vi "New JSON Numeric.vi"(8 "error in (no error)":errorcluster, 10 "value":dbl) -> (0 "error out":errorcluster, 3 "JSON Value out":refnum<class "JSON Value.lvclass">)   [LabVIEW 2016, in "JSON Value.lvclass"]
doc: "Create a new JSON Numeric with the given value."
uses:
  JSON Value.lvclass
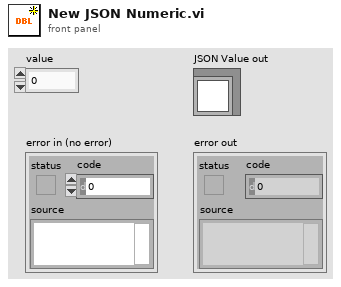
[diagram p1: front panel]
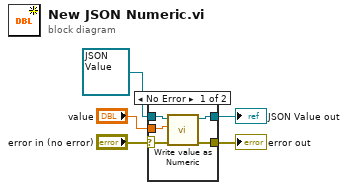
[diagram p0: block diagram]
diagram:
  n1 = case shown="No Error" "error in (no error)" {
    selector: "error in (no error)" -> [w8 w12]
    tunnel: [w10 w12] -> w4
    tunnel: [w6 w11] -> w3
    tunnel: refnum<class "JSON Value.lvclass"> refnum ("JSON out") -> [w9 w11]
    tunnel: "value" -> [w7 _]
    frame No Error {
      n2 = call "Write value as Numeric.vi"("error in (no error)"=w8, "value"=w7, "JSON Value in"=w9) -> ("error out"=w10:errorcluster, "JSON Value out"=w6:refnum<class "JSON Value.lvclass">)  [unwired: 7 in]
    }
    frame Error {
    }
  }
  "error out" <- w4
  "JSON Value out" <- w3
